vi "Entradas&Salidas.vi"() -> ()   [LabVIEW 2023]
uses:
  <vilib>/Instr/_visa.llb/VISA Configure Serial Port (Instr).vi
panel:
  in  "stop":bool
  in  "VISA resource name":refnum<visa-resource-name>
  out "BOTON 4":bool
  out "BOTON 3":bool
  out "BOTON 2":bool
  out "BOTON 1":bool
  in  "LED 4":bool
  in  "LED 3":bool
  in  "LED 2":bool
  in  "LED 1":bool
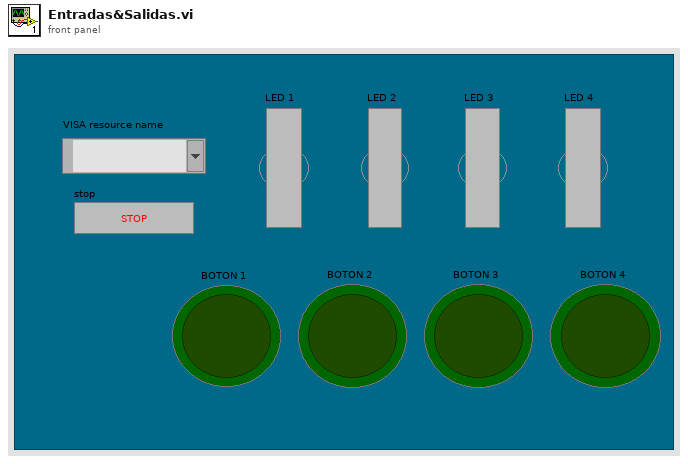
[diagram p1: front panel]
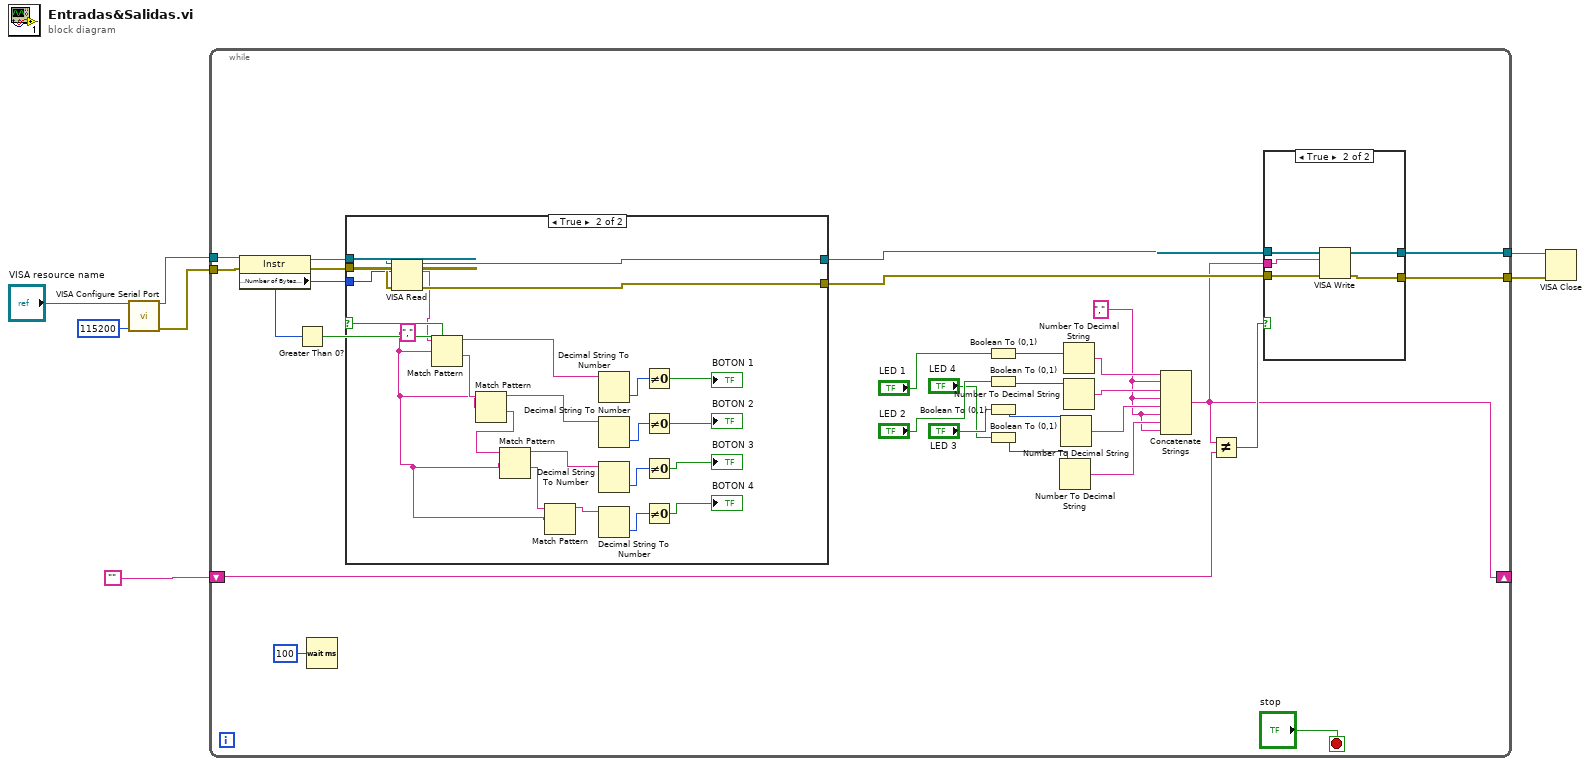
[diagram p0: block diagram]
diagram:
  n1 = call-poly "VISA Configure Serial Port"("VISA resource name"="VISA resource name", "baud rate (9600)"=u32 115200) -> ("VISA resource name out"=w6:refnum<visa-resource-name>, "error out"=w5:errorcluster)  [unwired: 12 in]
  n2 = while {
    tunnel: w6 -> [w35]
    tunnel: w5 -> [w34]
    tunnel: [w31] -> w3
    tunnel: [w28] -> w2
    shift-right: [w8] -> _
    shift-left: "" -> [w14]
    stop <- "stop" stop-if-true
    w15 = ","
    n3 = property class="Instr"(reference=w35, error in=w34) -> (reference out=w33:refnum<visa-resource-name>, error out=w29:errorcluster, "Serial Settings:Number of Bytes at Serial Port"=w24:u32)
    n4 = Greater Than 0?(x=w24) -> (x > 0?=w26:bool)
    n5 = Wait (ms)(milliseconds to wait=u32 100) -> ()  [unwired: 1 out]
    n6 = case shown="True" w26 {
      tunnel: w33 -> [w43 w66]
      tunnel: [w43 w65] -> w32
      tunnel: [w44 w64] -> w30
      tunnel: w29 -> [w44 w63]
      tunnel: w24 -> [_ w45]
      frame False {
      }
      frame True {
        w52 = "," ("regular expression")
        n7 = VISA Read(VISA resource name=w66, byte count=w45, error in (no error)=w63) -> (VISA resource name out=w65:refnum<visa-resource-name>, read buffer=w50:string, error out=w64:errorcluster)  [unwired: 1 out]
        n8 = Match Pattern(string=w50, regular expression=w52) -> (before substring=w62:string, after substring=w60:string)  [unwired: 1 in, 2 out]
        n9 = Match Pattern(string=w60, regular expression=w52) -> (before substring=w58:string, after substring=w54:string)  [unwired: 1 in, 2 out]
        n10 = Match Pattern(string=w54, regular expression=w52) -> (before substring=w55:string, after substring=w53:string)  [unwired: 1 in, 2 out]
        n11 = Match Pattern(string=w53, regular expression=w52) -> (before substring=w51:string)  [unwired: 1 in, 3 out]
        n12 = Decimal String To Number(string=w62) -> (number=w61:i32)  [unwired: 2 in, 1 out]
        n13 = Decimal String To Number(string=w58) -> (number=w59:i32)  [unwired: 2 in, 1 out]
        n14 = Decimal String To Number(string=w55) -> (number=w57:i32)  [unwired: 2 in, 1 out]
        n15 = Decimal String To Number(string=w51) -> (number=w56:i32)  [unwired: 2 in, 1 out]
        n16 = Not Equal To 0?(x=w61) -> (x != 0?=→"BOTON 1":bool)
        n17 = Not Equal To 0?(x=w59) -> (x != 0?=→"BOTON 2":bool)
        n18 = Not Equal To 0?(x=w57) -> (x != 0?=→"BOTON 3":bool)
        n19 = Not Equal To 0?(x=w56) -> (x != 0?=→"BOTON 4":bool)
      }
    }
    n20 = Boolean To (0,1)(Boolean="LED 1") -> (0, 1=w23:i16)
    n21 = Boolean To (0,1)(Boolean="LED 2") -> (0, 1=w22:i16)
    n22 = Boolean To (0,1)(Boolean="LED 3") -> (0, 1=w21:i16)
    n23 = Boolean To (0,1)(Boolean="LED 4") -> (0, 1=w20:i16)
    n24 = Number To Decimal String(number=w20) -> (decimal integer string=w16:string)  [unwired: 1 in]
    n25 = Number To Decimal String(number=w21) -> (decimal integer string=w17:string)  [unwired: 1 in]
    n26 = Number To Decimal String(number=w23) -> (decimal integer string=w19:string)  [unwired: 1 in]
    n27 = Number To Decimal String(number=w22) -> (decimal integer string=w18:string)  [unwired: 1 in]
    n28 = Concatenate Strings(w19, w15, w18, w15, w17, w15, w16, w15) -> (w8:string)
    n29 = Not Equal?(x=w8, y=w14) -> (x != y?=w13:bool)
    n30 = case shown="True" w13 {
      tunnel: w32 -> [w37 w42]
      tunnel: [w37 w41] -> w31
      tunnel: w30 -> [w36 w40]
      tunnel: [w36 w39] -> w28
      tunnel: w8 -> [_ w38]
      frame False {
      }
      frame True {
        n31 = VISA Write(VISA resource name=w42, write buffer=w38, error in (no error)=w40) -> (VISA resource name out=w41:refnum<visa-resource-name>, error out=w39:errorcluster)  [unwired: 1 out]
      }
    }
  }
  n32 = VISA Close(VISA resource name=w3, error in (no error)=w2) -> ()  [unwired: 1 out]
